vi "Find RT Module.vi"() -> (2 "RT Module Installed?":bool)   [LabVIEW 2026]
uses:
  <vilib>/nisyscfg/Get Installed Components.vi
  <vilib>/nisyscfg/nisyscfg.lvlib
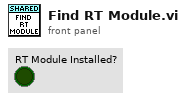
[diagram p1: front panel]
types:
  T1 = typedef "nisyscfg.lvlib/Software 1.2.ctl" = cluster{"title":string, "description":string, "ID":string, "version":string, "component type":T2}
  T2 = typedef "nisyscfg.lvlib/Component Type.ctl" = u32
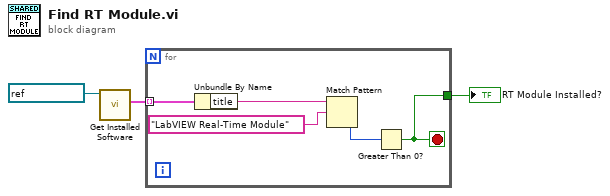
[diagram p0: block diagram]
diagram:
  n1 = call-poly <vilib>:"Get Installed Software.vi"("Session in"=refnum<k21> "localhost") -> ("Software Components"=w3:T1[])  [unwired: 8 in, 2 out]
  n2 = for {
    tunnel: w3 -> [w7] mode=indexing
    tunnel: [w4] -> w2
    stop <- w4 stop-if-true
    n3 = Unbundle By Name(w7) -> ("title"=w6:string)
    n4 = Match Pattern(string=w6, regular expression="LabVIEW Real-Time Module") -> (offset past match=w5:i32)  [unwired: 1 in, 3 out]
    n5 = Greater Than 0?(x=w5) -> (x > 0?=w4:bool)
  }
  "RT Module Installed?" <- w2
